vi "INI_Startup.vi"() -> (0 "PitchMin":dbl, 1 "PitchMax":dbl, 2 "PitchFiring":dbl, 3 "PitchLoading":dbl)   [LabVIEW 2012]
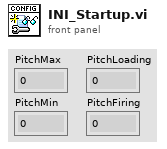
[diagram p1: front panel]
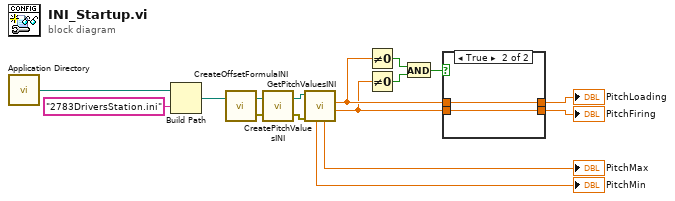
[diagram p0: block diagram]
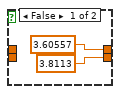
[diagram p2: hidden frame]
diagram:
  n1 = call <vilib>:"Application Directory.vi"() -> ("Application Directory"=w16:path)
  n2 = Build Path(base path=w16, name or relative path="2783DriversStation.ini") -> (appended path=w14:path)
  n3 = call "CreateOffsetFormulaINI.vi"("configuration file path"=w14) -> ("error out"=w12:errorcluster, "file path"=w13:path)  [unwired: 1 in]
  n4 = call "CreatePitchValuesINI.vi"("error in (no error)"=w12, "configuration file path"=w13) -> ("error out"=w10:errorcluster, "file path"=w11:path)
  n5 = call "GetPitchValuesINI.vi"("error in (no error)"=w10, "configuration file path"=w11) -> ("PitchFiring"=w5:dbl, "PitchLoading"=w6:dbl, "PitchMax"=→"PitchMax":dbl, "PitchMin"=→"PitchMin":dbl)  [unwired: 4 in, 2 out]
  n6 = Not Equal To 0?(x=w6) -> (x != 0?=w9:bool)
  n7 = Not Equal To 0?(x=w5) -> (x != 0?=w8:bool)
  n8 = And(x=w9, y=w8) -> (x .and. y?=w7:bool)
  n9 = case shown="True" w7 {
    tunnel: w6 -> [_ w20]
    tunnel: w5 -> [_ w19]
    tunnel: [3.60557 ("Value (Signaling)") w20] -> w4
    tunnel: [3.8113 ("Value (Signaling)") w19] -> w3
    frame False {
    }
    frame True {
    }
  }
  "PitchLoading" <- w4
  "PitchFiring" <- w3
